vi "Main.vi"(8 "error in (no error)":errorcluster, 11 "ModuleAdmin":refnum<class "ModuleAdmin.lvclass">) -> ()   [LabVIEW 2014, in "SamplerModule.lvlib"]
uses:
  SamplerModule.lvlib
  <userlib>/NIST/ModuleAdminLib/ModuleAdmin/ModuleAdmin.lvclass
  PublicAPI/Arguments/Requests/clStopArgument.ctl
  SamplerPlugins/NISTSamplerPluginsBaseClass/SamplerPluginsBase.lvclass
  <userlib>/NIST/ModuleAdminLib/ModuleAdmin/ModuleAdmin.lvclass/ModuleAdmin.ctl
  <userlib>/NIST/BaseClasses/BasePlugin_class/BasePlugin.lvclass/BasePlugin.ctl
  SamplerPlugins/NISTSamplerPluginsBaseClass/TypeDefs/ConfigMeasurementParams.ctl
  SamplerPlugins/NISTSamplerPluginsBaseClass/TypeDefs/ConfigTriggerParams.ctl
  SamplerPlugins/NISTSamplerPluginsBaseClass/TypeDefs/ConfigACBandwidthParams.ctl
  SamplerPlugins/NISTSamplerPluginsBaseClass/TypeDefs/ConfigMultiPointParams.ctl
  SamplerPlugins/NISTSamplerPluginsBaseClass/TypeDefs/MultiPointParams.ctl
  SamplerPlugins/NISTSamplerPluginsBaseClass/TypeDefs/CorrectionFactors.ctl
  SamplerPlugins/NISTSamplerPluginsBaseClass/SamplerPluginsBase.lvclass/SamplerPluginsBase.ctl
  <vilib>/Utility/error.llb/DialogType.ctl
  <userlib>/NIST/ModuleAdminLib/ModuleAdmin/Accessors/Read ShowPanel_.vi
  <userlib>/NIST/BaseClasses/BasePlugin_class/Accessors/Write PluginIniFilePath.vi
  <userlib>/NIST/BaseClasses/BasePlugin_class/Accessors/Read PluginIniFilePath.vi
  SamplerPlugins/NISTSamplerPluginsBaseClass/Accessors/Write CorrectionFactors.vi
  SamplerPlugins/NISTSamplerPluginsBaseClass/Accessors/Read CorrectionFactors.vi
  <userlib>/NIST/ModuleAdminLib/ModuleAdmin/Accessors/Write ShowPanel_.vi
  <userlib>/NIST/ModuleAdminLib/ModuleAdmin/Accessors/Read CloneRegRef.vi
  <vilib>/Utility/error.llb/Error Cluster From Error Code.vi
  <vilib>/ErrorRing/Error Ring.xnode
  <userlib>/NIST/ModuleAdminLib/CloneRegistration/CloneRegistration.lvclass
  <userlib>/NIST/ModuleAdminLib/ModuleAdmin.lvlib
  <userlib>/NIST/BaseClasses/Object_class/BaseObject.lvclass
panel:
  out "error out":errorcluster
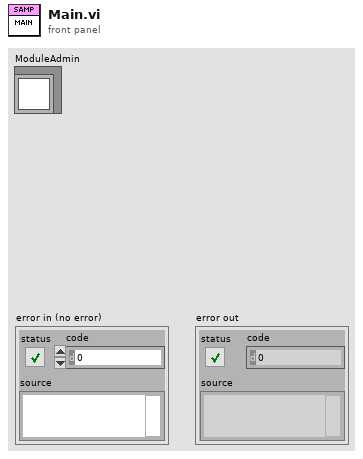
[diagram p1: front panel]
types:
  T1 = typedef "SamplerModule.lvlib/clRequestEvents.ctl" = cluster{"StopRequest":refnum<user-event>, "PathToINI":refnum<user-event>, " LoadPlugin":refnum<user-event>, "ConfigMeasurement":refnum<user-event>, "Read":refnum<user-event>, "GetReading":refnum<user-event>, "InitializeDevice":refnum<user-event>, "ResetRequest":refnum<user-event>, "AbortRequest":refnum<user-event>, "FetchRequest":refnum<user-event>, "InitiateRequest":refnum<user-event>, "ConfigTrigger":refnum<user-event>, "IsOverRange":refnum<user-event>, "ConfigACBandwidth":refnum<user-event>, "ConfigFreqVoltRange":refnum<user-event>, "ConfigMeasCompDest":refnum<user-event>, "FetchMultiPoint":refnum<user-event>, "ReadMultiPoint":refnum<user-event>, "ConfigMultiPoint":refnum<user-event>, "GetMultiPointReading":refnum<user-event>, "InitiateMultiPoint":refnum<user-event>, "ShowPanel":refnum<user-event>, "WriteMultiPointParams":refnum<user-event>, "EvtSignal":refnum<user-event>, "ReadMultiPointParams":refnum<user-event>, "ReadMultiPointConfig":refnum<user-event>, "WriteMultiPointConfig":refnum<user-event>, "ReadCorrFactors":refnum<user-event>, "Write CorrFactors":refnum<user-event>, "ConfigDialog":refnum<user-event>}
  T2 = typedef "SamplerModule.lvlib/clBroadcastEvents.ctl" = cluster{"DidInit":refnum<user-event>, "StatusUpdate":refnum<user-event>, "ErrorReport":refnum<user-event>, "DidStop":refnum<user-event>, "PathToINI":refnum<user-event>, "GetReading":refnum<user-event>, "IsOverRange":refnum<user-event>, "GetMultiPointReading":refnum<user-event>, "MultiPointParams":refnum<user-event>, "MultiPointConfig":refnum<user-event>, "CorrFactors":refnum<user-event>}
  T3 = typedef "SamplerModule.lvlib/clStopArgument.ctl" = cluster{"Exit via Stop Module Req?":bool, "Wait for Module to stop?":bool, "ModuleAdmin":refnum<class "ModuleAdmin.lvclass">}
  T4 = enum32{"Invalid", "Standard", "Closed", "Hidden", "Minimized", "Maximized"}
  T5 = typedef "SamplerPlugins.lvlib/SamplerPluginsBase.lvclass/ConfigMeasurementParams.ctl" = cluster{"eFunction":u16, "dRange":dbl, "dResolution":dbl}
  T6 = typedef "SamplerPlugins.lvlib/SamplerPluginsBase.lvclass/ConfigTriggerParams.ctl" = cluster{"eTriggerSource":u16, "dTriggerDelay":dbl}
  T7 = typedef "SamplerPlugins.lvlib/SamplerPluginsBase.lvclass/ConfigACBandwidthParams.ctl" = cluster{"dMinFreq":dbl, "dMaxFreq":dbl}
  T8 = typedef "SamplerPlugins.lvlib/SamplerPluginsBase.lvclass/ConfigMultiPointParams.ctl" = cluster{"iTriggerCount":i32, "iSampleCount":i32, "eSampleClock":u16, "dSampleInterval":dbl}
  T9 = typedef "SamplerPlugins.lvlib/SamplerPluginsBase.lvclass/MultiPointParams.ctl" = cluster{"iMaxTimeMilliseconds":i32, "iArraySize":i32}
  T10 = typedef "SamplerPlugins.lvlib/SamplerPluginsBase.lvclass/CorrectionFactors.ctl" = cluster{"MagCorr":dbl[], "DlyCorr":dbl[]}
  T11 = typedef "SamplerPlugins.lvlib/SamplerPluginsBase.lvclass/MultiPointReadingArrayParams.ctl" = T12[]
  T12 = typedef "SamplerPlugins.lvlib/SamplerPluginsBase.lvclass/MultiPointReadingParams.ctl" = cluster{"dReadingArray":dbl[], "iActualPts":i32, "Timestamp":dbl}
  T13 = typedef "DialogType.ctl" = u16
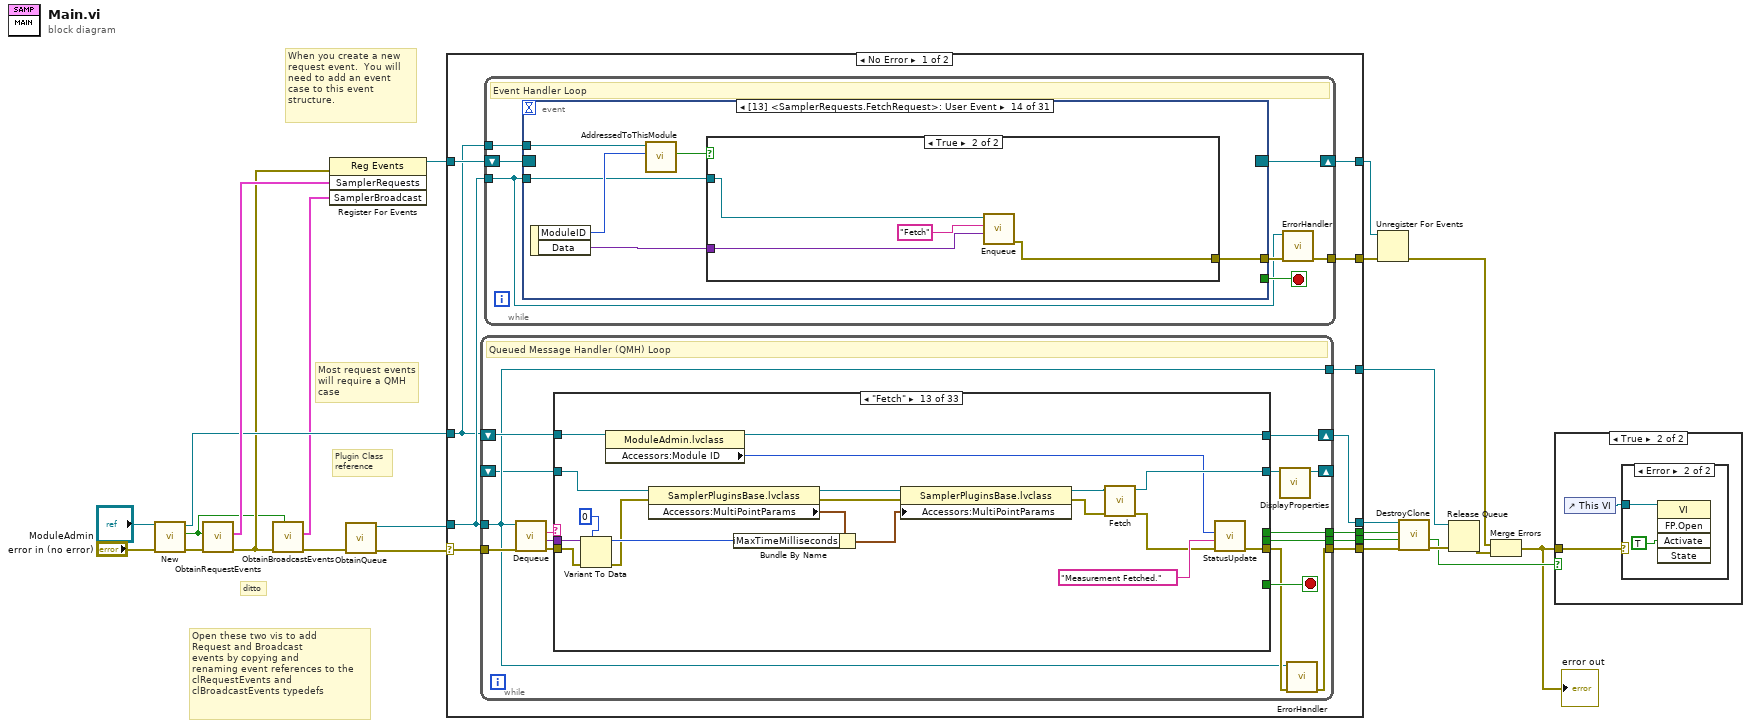
[diagram p0: block diagram]
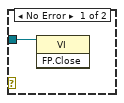
[diagram p3: hidden frame]
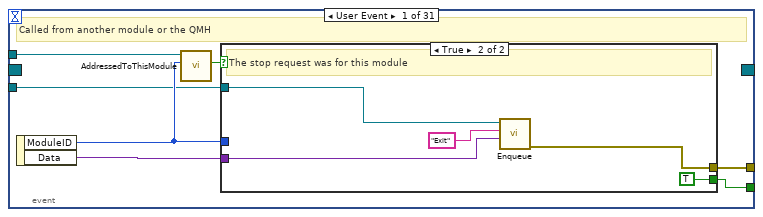
[diagram p4: hidden frame]
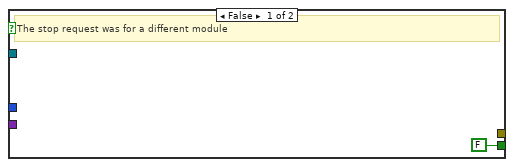
[diagram p5: hidden frame]
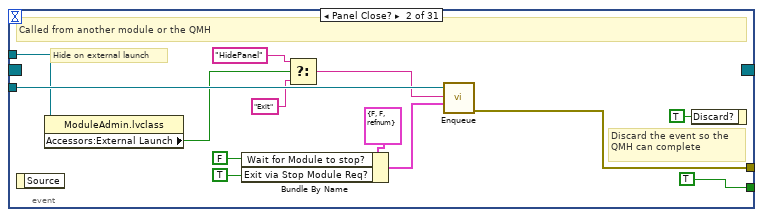
[diagram p6: hidden frame]
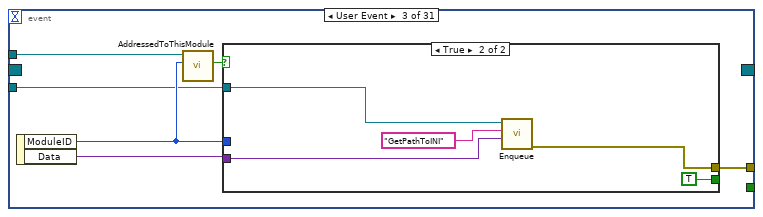
[diagram p7: hidden frame]
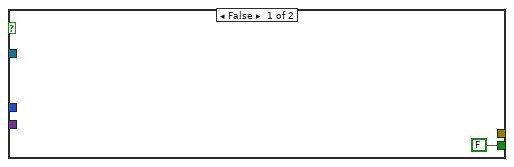
[diagram p8: hidden frame]
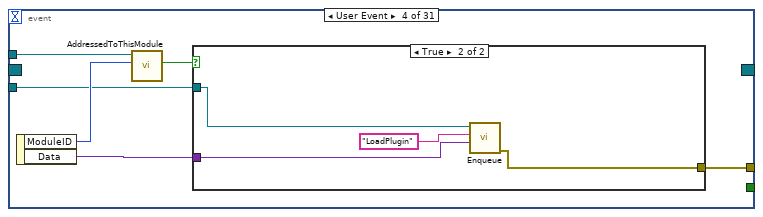
[diagram p9: hidden frame]
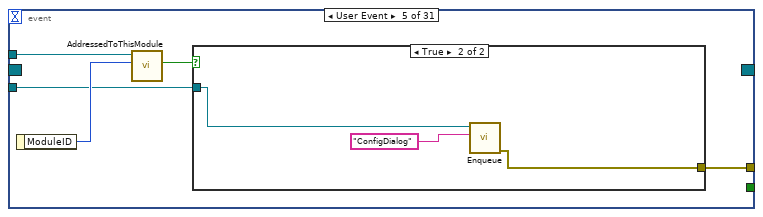
[diagram p11: hidden frame]
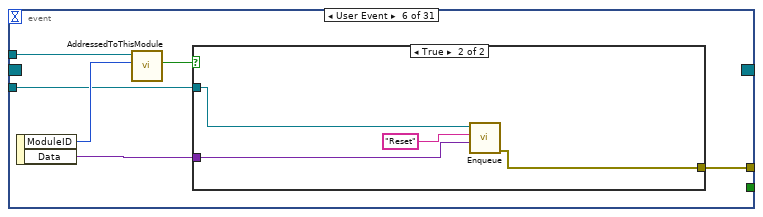
[diagram p13: hidden frame]
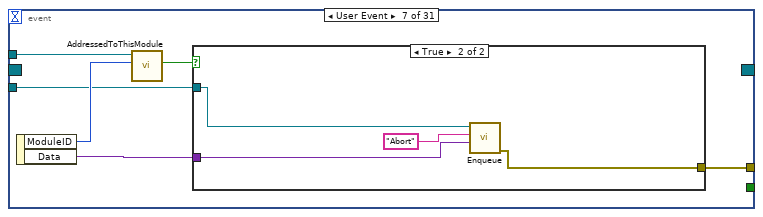
[diagram p15: hidden frame]
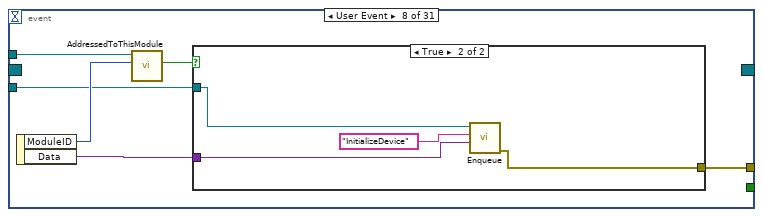
[diagram p17: hidden frame]
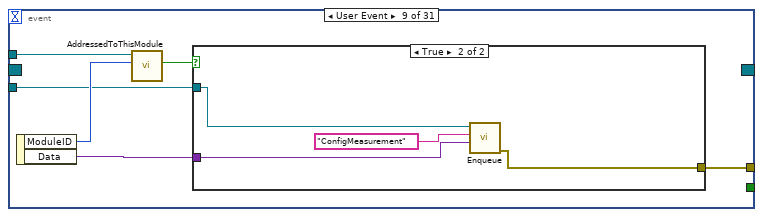
[diagram p19: hidden frame]
diagram:
  # "Plugin Class\nreference"
  # "Open these two vis to add\nRequest and Broadcast \nevents by copying and \nrenaming event references to the \nclRequestEvents and \nclBroadcastEvents typedefs"
  # "ditto"
  # "Most request events\nwill require a QMH\ncase"
  # "When you create a new request event.  You will need to add an event case to this event structure."
  n1 = call <userlib>:"New.vi"("error in (no error)"="error in (no error)", "ModuleAdmin"="ModuleAdmin") -> ("error out"=w22:errorcluster, "First?"=w1:bool, "ModuleAdmin"=w18:refnum<class "ModuleAdmin.lvclass">)  [unwired: 7 in]
  n2 = call "ObtainRequestEvents.vi"("error in (no error)"=w22, "CreateNew (f)"=w1) -> ("error out"=w15:errorcluster, "SamplerRequests"=w21:T1)  [unwired: 8 in]
  n3 = call "ObtainBroadcastEvents.vi"("Init? (f)"=w1, "error in (no error)"=w15) -> ("error out"=w16:errorcluster, "SamplerBroadcast"=w14:T2)  [unwired: 8 in]
  n4 = register-events(error in=w15, w21, w14) -> (reference out=w13:refnum<event-registration>)  [unwired: 1 in, 1 out]
  n5 = call "ObtainQueue.vi"("error in (no error)"=w16) -> ("error out"=w20:errorcluster, "MessageQueue"=w19:refnum<queue>)  [unwired: 9 in]
  n6 = case shown="No Error" w20 {
    selector: w20 -> [w35 w866]
    tunnel: w19 -> [w33 w862]
    tunnel: w18 -> [w30 w863]
    tunnel: [w34 w864] -> w12
    tunnel: [w32 w862] -> w17
    tunnel: w13 -> [w31 w858]
    tunnel: [w29 w861] -> w10
    tunnel: [w28 _] -> w9
    tunnel: [w27 _] -> w8
    tunnel: [w26 _] -> w5
    tunnel: [w25 w858] -> w4
    frame No Error {
      n7 = while {
        tunnel: w33 -> [w361]
        tunnel: w35 -> [w370]
        tunnel: [w363] -> w34
        tunnel: [w361] -> w32
        tunnel: [w365] -> w28
        tunnel: [w364] -> w27
        shift-right: [w358] -> _
        shift-left: _ -> [w360]
        shift-right: [w357] -> w29
        shift-left: w30 -> [w366]
        stop <- w371 stop-if-true
        # "Queued Message Handler (QMH) Loop"
        n8 = call "Dequeue.vi"("error in (no error)"=w370, "MessageQueue"=w361) -> ("error out"=w369:errorcluster, "Message Data"=w367:variant, "Message"=w368:string)  [unwired: 6 in, 1 out]
        n9 = case shown="\"Fetch\"" w368 {
          selector: w368 -> [w376 _ _ _ _ _ _ _ _ _ _ _ _ _ _ _ _ _ _ _ _ _ _ _ _ _ _ _ _ _ _ _ _]
          tunnel: [_ _ _ _ _ _ _ _ _ _ _ _ _ _ TRUE _ _ _ _ _ _ _ _ _ _ _ _ _ _ _ _ _ _] -> w371
          tunnel: w366 -> [w379 w408 w425 w434 w443 w453 w493 w503 w524 w542 w557 w572 w592 w604 w605 w625 w648 w659 w675 w686 w702 w717 w730 w747 w756 w765 w785 w798 w810 w820 w830 w839 w848]
          tunnel: [w375 w397 w424 w433 w442 w454 w492 w501 w523 w541 w556 w571 w591 w603 w614 w626 w649 w655 w668 w684 w701 w716 w729 w746 w755 w764 w784 w797 w803 w814 w824 w836 w851] -> w362
          tunnel: w369 -> [_ _ w421 w431 w440 w458 w496 w512 w530 w545 w560 w575 w594 w600 w607 w634 w644 w656 w672 w678 w705 w720 w726 w742 w751 w768 w788 w801 w811 w821 w831 w843 w849]
          tunnel: w367 -> [_ _ _ _ _ w460 _ w513 w531 w546 w561 w576 w595 _ w613 w633 _ _ _ _ w706 w721 _ _ _ w769 w789 w802 _ _ _ w845 w850]
          tunnel: [_ _ _ _ _ _ _ _ _ _ _ _ _ _ w611 _ _ _ _ _ _ _ _ _ _ _ _ _ _ _ _ _ _] -> w365
          tunnel: [_ _ _ _ _ _ _ _ _ _ _ _ _ _ w610 _ _ _ _ _ _ _ _ _ _ _ _ _ _ _ _ _ _] -> w364
          tunnel: [w373 refnum<class "SamplerPluginsBase.lvclass"> refnum ("MyPlugins.lvlib:MyPluginsBase.lvclass") w423 w430 w441 w451 w494 w502 w521 w540 w555 w568 w587 w601 w608 w624 w645 w657 w673 w685 w688 w711 w727 w740 w754 w761 w781 w794 w805 w816 w826 w840 w846] -> w359
          tunnel: w360 -> [w373 _ w422 w432 w439 w452 w495 w511 w529 w544 w559 w574 w593 w602 w609 w624 w647 w658 w674 w680 w704 w719 w728 w743 w753 w767 w787 w800 w812 w822 w832 w842 w846]
          tunnel: [w372 w392 w420 w429 w438 w450 w493 w500 w518 w535 w550 w565 w586 w599 w605 w622 w642 w651 w670 w676 w687 w710 w725 w744 w752 w760 w780 w793 w806 w817 w827 w838 w847] -> w357
          frame Default {
            # "Called only if a message was queued and no QMH case was created"
            n10 = property class="ModuleAdmin.lvclass"(reference=w379) -> (reference out=w372:refnum<class "ModuleAdmin.lvclass">, "Accessors:Module ID"=w378:i32, "Accessors:ModuleName"=w374:string)  [unwired: 1 in, 1 out]
            n11 = call <userlib>:"ModuleName.vi"("Name"=w374, "ModuleID"=w378) -> ("ModuleName"=w377:string)  [unwired: 9 in]
            n12 = xnode "Error Ring"("parameter 0"=w376, "parameter 1"=w377) -> ("error out"=w375:errorcluster)
          }
          frame "Initialize" {
            # "Initialize is always called after ObtainQueue.vi is run"
            n13 = property class="ModuleAdmin.lvclass"(reference=w408) -> (reference out=w394:refnum<class "ModuleAdmin.lvclass">, error out=w405:errorcluster, "Accessors:Module ID"=w396:i32, "Accessors:ShowPanel_"=w391:bool, "Accessors:External Launch"=w389:bool, "Accessors:ModuleName"=w388:string)  [unwired: 1 in]
            n14 = Compound Arithmetic op=OR(w391, invert w389) -> (w390:bool)
            n15 = Select(t=T4."Standard" ("Front Panel Window:State"), s=w390, f=T4."Hidden" ("Front Panel Window:State")) -> (s? t:f=w401:T4)
            n16 = invoke class="VI" method="FP.Open"(error in=w405, "State"=w401) -> (error out=w404:errorcluster)  [unwired: 3 in, 4 out]
            n17 = call <userlib>:"ModuleName.vi"("Name"=w388, "ModuleID"=w396) -> ("ModuleName"=w400:string)  [unwired: 9 in]
            n18 = property class="VI"(error in=w404, "Front Panel.Title"=w400) -> (reference out=w407:refnum<vi>, error out=w406:errorcluster)  [unwired: 1 in]
            n19 = invoke class="VI" method="FP.Center"(reference=w407, error in=w406) -> (error out=w395:errorcluster)  [unwired: 1 in, 2 out]
            n20 = case shown="True" w389 {
              tunnel: [w409 w415] -> w398
              tunnel: [w410 w412] -> w392
              tunnel: w395 -> [w409 w414]
              tunnel: w394 -> [w410 w411]
              frame False {
              }
              frame True {
                n21 = call <userlib>:"WaitOnModuleSync.vi"("error in (no error)"=w414, "ModuleAdmin"=w411) -> ("error out"=w416:errorcluster, "ModuleAdmin"=w413:refnum<class "ModuleAdmin.lvclass">)  [unwired: 8 in]
                n22 = call <userlib>:"WaitOnEventSync.vi"("error in (no error)"=w416, "ModuleAdmin"=w413) -> ("error out"=w415:errorcluster, "ModuleAdmin"=w412:refnum<class "ModuleAdmin.lvclass">)  [unwired: 8 in]
              }
            }
            n23 = call "DidInit.vi"("Init?"=TRUE, "error in (no error)"=w398, "ModuleAdmin"=w392) -> ("error out"=w397:errorcluster)  [unwired: 8 in]
          }
          frame "Reset" {
            n24 = property class="ModuleAdmin.lvclass"(reference=w425) -> (reference out=w420:refnum<class "ModuleAdmin.lvclass">, "Accessors:Module ID"=w417:i32)  [unwired: 1 in, 1 out]
            n25 = call-dynamic "Reset.vi"("error in (no error)"=w421, "NISTSamplerPluginsBase in"=w422) -> ("error out"=w418:errorcluster, "NISTSamplerPluginsBase out"=w423:refnum<class "SamplerPluginsBase.lvclass">)  [unwired: 8 in]
            n26 = call "StatusUpdate.vi"("error in (no error)"=w418, "Status"="Device is reset.", "ModuleID"=w417) -> ("error out"=w424:errorcluster)  [unwired: 8 in]
          }
          frame "Abort" {
            n27 = property class="ModuleAdmin.lvclass"(reference=w434) -> (reference out=w429:refnum<class "ModuleAdmin.lvclass">, "Accessors:Module ID"=w427:i32)  [unwired: 1 in, 1 out]
            n28 = call-dynamic "Abort.vi"("error in (no error)"=w431, "NISTSamplerPluginsBase in"=w432) -> ("error out"=w428:errorcluster, "NISTSamplerPluginsBase out"=w430:refnum<class "SamplerPluginsBase.lvclass">)  [unwired: 8 in]
            n29 = call "StatusUpdate.vi"("error in (no error)"=w428, "Status"="Operation Aborted.", "ModuleID"=w427) -> ("error out"=w433:errorcluster)  [unwired: 8 in]
          }
          frame "InitializeDevice" {
            # "Resets the device, clear tasks, creates new task, sets trigger and clock"
            n30 = property class="ModuleAdmin.lvclass"(reference=w443) -> (reference out=w438:refnum<class "ModuleAdmin.lvclass">, "Accessors:Module ID"=w437:i32)  [unwired: 1 in, 1 out]
            n31 = call-dynamic "InitializeDevice.vi"("error in (no error)"=w440, "NISTSamplerPluginsBase in"=w439) -> ("error out"=w435:errorcluster, "NISTSamplerPluginsBase out"=w441:refnum<class "SamplerPluginsBase.lvclass">)  [unwired: 8 in]
            n32 = call "StatusUpdate.vi"("error in (no error)"=w435, "Status"="Device is initialized.", "ModuleID"=w437) -> ("error out"=w442:errorcluster)  [unwired: 8 in]
          }
          frame "LoadPlugin" {
            n33 = Variant To Data(error in=w458, type=path "", Variant=w460) -> (data=w448:path, error out=w449:errorcluster)
            n34 = call <userlib>:"GetPathToClass.vi"("error in (no error)"=w449, "configuration file path"=w448) -> ("error IO"=w445:errorcluster, "PathToClass"=w447:path)  [unwired: 8 in]
            n35 = Current VI's Path() -> (path=w446:path)
            n36 = Build Path(base path=w446, name or relative path=w447) -> (appended path=w444:path)
            n37 = call <vilib>:"Check if File or Folder Exists.vi"("error in (no error)"=w445, "path"=w444) -> ("error out"=w455:errorcluster, "file or folder exists?"=w457:bool, "dup path"=w456:path)  [unwired: 7 in]
            n38 = case shown="True" w457 {
              tunnel: w456 -> [w466 w483]
              tunnel: w455 -> [w464 w491]
              tunnel: [w462 w486] -> w454
              tunnel: w453 -> [w461 w485]
              tunnel: w452 -> [w465 _]
              tunnel: [w465 w476] -> w451
              tunnel: w448 -> [_ w482]
              tunnel: [w461 w481] -> w450
              frame False {
                n39 = Path To String(path=w466) -> (string=w467:string)
                n40 = xnode "Error Ring"("parameter 0"=w467) -> ("error out"=w463:errorcluster)
                n41 = Merge Errors(w464, w463) -> (w462:errorcluster)
              }
              frame True {
                n42 = call-dynamic "LoadClassFromFile.vi"("error in (no error)"=w491, "class path"=w483, "reference in"=refnum<class "SamplerPluginsBase.lvclass"> refnum ("MyPlugins.lvlib:MyPluginsBase.lvclass")) -> ("error out"=w480:errorcluster, "reference out"=w479:refnum<class "SamplerPluginsBase.lvclass">)  [unwired: 7 in]
                n43 = property class="SamplerPluginsBase.lvclass"(reference=w479, error in=w480, "Accessors:PluginIniFilePath"=w482) -> (reference out=w478:refnum<class "SamplerPluginsBase.lvclass">, error out=w477:errorcluster)
                n44 = property class="ModuleAdmin.lvclass"(reference=w485) -> (reference out=w481:refnum<class "ModuleAdmin.lvclass">, "Accessors:Module ID"=w484:i32)  [unwired: 1 in, 1 out]
                n45 = Path To String(path=w483) -> (string=w488:string)
                n46 = Format Into String(format string="Plugin %s loaded ", w488) -> (resulting string=w487:string)  [unwired: 2 in, 1 out]
                n47 = call-dynamic "DefaultFromIni.vi"("error in (no error)"=w477, "SamplerPluginsBase in"=w478) -> ("error out"=w475:errorcluster, "SamplerPluginsBase out"=w476:refnum<class "SamplerPluginsBase.lvclass">)  [unwired: 8 in]
                n48 = call "StatusUpdate.vi"("error in (no error)"=w475, "Status"=w487, "ModuleID"=w484) -> ("error out"=w486:errorcluster)  [unwired: 8 in]
              }
            }
          }
          frame "ConfigDialog" {
            n49 = call-dynamic "ConfigDialog.vi"("error in (no error)"=w496, "SamplerPluginsBase in"=w495) -> ("error out"=w492:errorcluster, "SamplerPluginsBase out"=w494:refnum<class "SamplerPluginsBase.lvclass">)  [unwired: 8 in]
          }
          frame "ConfigMeasurement" {
            n50 = Variant To Data(error in=w512, type=T5 {"eFunction"=0, "dRange"=0.0, "dResolution"=0.0} ("ConfigMeasurement"), Variant=w513) -> (data=w510:T5, error out=w505:errorcluster)
            n51 = property class="ModuleAdmin.lvclass"(reference=w503) -> (reference out=w500:refnum<class "ModuleAdmin.lvclass">, "Accessors:Module ID"=w497:i32)  [unwired: 1 in, 1 out]
            n52 = Unbundle By Name(w510) -> ("eFunction"=w509:u16, "dRange"=w508:dbl, "dResolution"=w507:dbl)
            n53 = property class="SamplerPluginsBase.lvclass"(reference=w511, error in=w505, "Accessors:eFunction"=w509, "Accessors:dRange"=w508, "Accessors:dResolution"=w507) -> (reference out=w506:refnum<class "SamplerPluginsBase.lvclass">, error out=w504:errorcluster)
            n54 = call-dynamic "ConfigMeasurement.vi"("error in (no error)"=w504, "NISTSamplerPluginsBase in"=w506) -> ("error out"=w499:errorcluster, "NISTSamplerPluginsBase out"=w502:refnum<class "SamplerPluginsBase.lvclass">)  [unwired: 8 in]
            n55 = call "StatusUpdate.vi"("error in (no error)"=w499, "Status"="Measurement Configured." ("input 3"), "ModuleID"=w497) -> ("error out"=w501:errorcluster)  [unwired: 8 in]
          }
          frame "ConfigTrigger" {
            n56 = Variant To Data(error in=w530, type=T6 {"eTriggerSource"=0, "dTriggerDelay"=0.0} ("ConfigTriggerParams"), Variant=w531) -> (data=w528:T6, error out=w525:errorcluster)
            n57 = property class="ModuleAdmin.lvclass" props=["Accessors:Module ID", "Accessors:Module ID"](reference=w524) -> (reference out=w518:refnum<class "ModuleAdmin.lvclass">, "Accessors:Module ID"=w517:i32)  [unwired: 1 in, 2 out]
            n58 = Unbundle By Name(w528) -> ("eTriggerSource"=w527:u16, "dTriggerDelay"=w526:dbl)
            n59 = property class="SamplerPluginsBase.lvclass"(reference=w529, error in=w525, "Accessors:eTriggerSource"=w527, "Accessors:dTriggerDelay"=w526) -> (reference out=w520:refnum<class "SamplerPluginsBase.lvclass">, error out=w519:errorcluster)
            n60 = call-dynamic "ConfigTrigger.vi"("error in (no error)"=w519, "NISTSamplerPluginsBase in"=w520) -> ("error out"=w516:errorcluster, "NISTSamplerPluginsBase out"=w521:refnum<class "SamplerPluginsBase.lvclass">)  [unwired: 8 in]
            n61 = call "StatusUpdate.vi"("error in (no error)"=w516, "Status"="Trigger Configured." ("input 3"), "ModuleID"=w517) -> ("error out"=w523:errorcluster)  [unwired: 8 in]
          }
          frame "ConfigACBandwidth" {
            n62 = Variant To Data(error in=w545, type=T7 {"dMinFreq"=0.0, "dMaxFreq"=0.0} ("ConfigACBandwidthParams"), Variant=w546) -> (data=w537:T7, error out=w543:errorcluster)
            n63 = property class="ModuleAdmin.lvclass"(reference=w542) -> (reference out=w535:refnum<class "ModuleAdmin.lvclass">, "Accessors:Module ID"=w534:i32)  [unwired: 1 in, 1 out]
            n64 = property class="SamplerPluginsBase.lvclass"(reference=w544, error in=w543, "Accessors:ConfigACBandwidthParams"=w537) -> (reference out=w539:refnum<class "SamplerPluginsBase.lvclass">, error out=w536:errorcluster)
            n65 = call-dynamic "ConfigACBandwidth.vi"("error in (no error)"=w536, "NISTSamplerPluginsBase in"=w539) -> ("error out"=w533:errorcluster, "NISTSamplerPluginsBase out"=w540:refnum<class "SamplerPluginsBase.lvclass">)  [unwired: 8 in]
            n66 = call "StatusUpdate.vi"("error in (no error)"=w533, "Status"="AC Bandwidth Configured." ("input 3"), "ModuleID"=w534) -> ("error out"=w541:errorcluster)  [unwired: 8 in]
          }
          frame "ConfigFreqVoltRange" {
            n67 = Variant To Data(error in=w560, type=0.0 ("dFrequencyVoltageRange"), Variant=w561) -> (data=w551:dbl, error out=w558:errorcluster)
            n68 = property class="ModuleAdmin.lvclass" props=["Accessors:Module ID", "Accessors:Module ID"](reference=w557) -> (reference out=w550:refnum<class "ModuleAdmin.lvclass">, "Accessors:Module ID"=w549:i32)  [unwired: 1 in, 2 out]
            n69 = property class="SamplerPluginsBase.lvclass"(reference=w559, error in=w558, "Accessors:dFrequencyVoltageRange"=w551) -> (reference out=w553:refnum<class "SamplerPluginsBase.lvclass">, error out=w554:errorcluster)
            n70 = call-dynamic "ConfigFreqVoltRange.vi"("error in (no error)"=w554, "NISTSamplerPluginsBase in"=w553) -> ("error out"=w548:errorcluster, "NISTSamplerPluginsBase out"=w555:refnum<class "SamplerPluginsBase.lvclass">)  [unwired: 8 in]
            n71 = call "StatusUpdate.vi"("error in (no error)"=w548, "Status"="Frequency Voltage Range Configured." ("input 3"), "ModuleID"=w549) -> ("error out"=w556:errorcluster)  [unwired: 8 in]
          }
          frame "Read" {
            n72 = Variant To Data(error in=w575, type=0 ("iMaxTimeMilliseconds"), Variant=w576) -> (data=w570:i32, error out=w573:errorcluster)
            n73 = property class="ModuleAdmin.lvclass"(reference=w572) -> (reference out=w565:refnum<class "ModuleAdmin.lvclass">, "Accessors:Module ID"=w564:i32)  [unwired: 1 in, 1 out]
            n74 = property class="SamplerPluginsBase.lvclass"(reference=w574, error in=w573, "Accessors:iMaxTimeMilliseconds"=w570) -> (reference out=w566:refnum<class "SamplerPluginsBase.lvclass">, error out=w567:errorcluster)
            n75 = call-dynamic "Read.vi"("error in (no error)"=w567, "NISTSamplerPluginsBase in"=w566) -> ("error out"=w562:errorcluster, "NISTSamplerPluginsBase out"=w568:refnum<class "SamplerPluginsBase.lvclass">)  [unwired: 8 in]
            n76 = call "StatusUpdate.vi"("error in (no error)"=w562, "Status"="Measurement Read." ("input 3"), "ModuleID"=w564) -> ("error out"=w571:errorcluster)  [unwired: 8 in]
          }
          frame "Fetch" {
            n77 = Variant To Data(error in=w594, type=0 ("iMaxTimeMilliseconds"), Variant=w595) -> (data=w582:i32, error out=w580:errorcluster)
            n78 = property class="ModuleAdmin.lvclass"(reference=w592) -> (reference out=w586:refnum<class "ModuleAdmin.lvclass">, "Accessors:Module ID"=w585:i32)  [unwired: 1 in, 1 out]
            n79 = property class="SamplerPluginsBase.lvclass"(reference=w593, error in=w580) -> (reference out=w581:refnum<class "SamplerPluginsBase.lvclass">, error out=w579:errorcluster, "Accessors:MultiPointParams"=w578:T9)
            n80 = Bundle By Name(cluster=w578, "iMaxTimeMilliseconds"=w582) -> (w577:T9)
            n81 = property class="SamplerPluginsBase.lvclass"(reference=w581, error in=w579, "Accessors:MultiPointParams"=w577) -> (reference out=w589:refnum<class "SamplerPluginsBase.lvclass">, error out=w588:errorcluster)
            n82 = call-dynamic "Fetch.vi"("error in (no error)"=w588, "NISTSamplerPluginsBase in"=w589) -> ("error out"=w583:errorcluster, "NISTSamplerPluginsBase out"=w587:refnum<class "SamplerPluginsBase.lvclass">)  [unwired: 8 in]
            n83 = call "StatusUpdate.vi"("error in (no error)"=w583, "Status"="Measurement Fetched." ("input 3"), "ModuleID"=w585) -> ("error out"=w591:errorcluster)  [unwired: 8 in]
          }
          frame "Initiate" {
            n84 = property class="ModuleAdmin.lvclass"(reference=w604) -> (reference out=w599:refnum<class "ModuleAdmin.lvclass">, "Accessors:Module ID"=w598:i32)  [unwired: 1 in, 1 out]
            n85 = call-dynamic "Initiate.vi"("error in (no error)"=w600, "NISTSamplerPluginsBase in"=w602) -> ("error out"=w596:errorcluster, "NISTSamplerPluginsBase out"=w601:refnum<class "SamplerPluginsBase.lvclass">)  [unwired: 8 in]
            n86 = call "StatusUpdate.vi"("error in (no error)"=w596, "Status"="Measurement Initiated.", "ModuleID"=w598) -> ("error out"=w603:errorcluster)  [unwired: 8 in]
          }
          frame "Exit" {
            # "Called by the StopRequest event handler case"
            n87 = disable-structure shown="Enabled" {
              disable-tunnel: w609 -> [w619 w621]
              disable-tunnel: [w618 w621] -> w608
              disable-tunnel: w607 -> [w617 w620]
              disable-tunnel: [w616 w620] -> w606
              frame Enabled {
                n88 = call-dynamic "CloseInstrumentSession.vi"("error in (no error)"=w617, "NISTSamplerPluginsBase in"=w619) -> ("error out"=w616:errorcluster, "NISTSamplerPluginsBase out"=w618:refnum<class "SamplerPluginsBase.lvclass">)  [unwired: 8 in]
              }
              frame Disabled {
              }
            }
            n89 = control-ref of="This VI"() -> (w612:refnum<vi>)
            n90 = call "HandleExit.vi"("error in (no error)"=w606, "VI Refnum"=w612, "StopArgument"=w613, "ModuleAdmin"=w605) -> ("error out"=w614:errorcluster, "Exit via Stop Module Req?"=w610:bool, "WaitForStop?"=w611:bool)  [unwired: 5 in]
          }
          frame "Error" {
            n91 = property class="ModuleAdmin.lvclass"(reference=w625) -> (reference out=w623:refnum<class "ModuleAdmin.lvclass">, "Accessors:External Launch"=w629:bool, "Accessors:Module ID"=w627:i32)  [unwired: 1 in, 1 out]
            n92 = Variant To Data(error in=w634, type=errorcluster {"status"=FALSE, "code"=0, "source"=""} ("error constant"), Variant=w633) -> (data=w628:errorcluster, error out=w631:errorcluster)
            n93 = call "ReportError.vi"("error in (no error)"=w631, "ErrorReported"=w628, "ModuleID"=w627) -> ("error out"=w630:errorcluster)  [unwired: 8 in]
            n94 = case shown="True" w629 {
              tunnel: w630 -> [w639 w641]
              tunnel: w628 -> [w638 _]
              tunnel: [w637 w641] -> w626
              tunnel: w625 -> [w636 _]
              tunnel: w623 -> [w635 w640]
              tunnel: [w635 w640] -> w622
              frame False {
                # "Todo:  Add an event to ask the user\nIf the module should stop or continue"
                # "Stand alone: now, force an exit"
                n95 = call <vilib>:"Simple Error Handler.vi"("error in (no error)"=w638) -> ()  [unwired: 4 in, 5 out]
                n96 = call "StopRequest.vi"("error in (no error)"=w639, "ModuleAdmin"=w636) -> ("error out"=w637:errorcluster)  [unwired: 8 in, 1 out]
              }
              frame True {
                # "Externally launched modules only broadcast the error msg"
              }
            }
          }
          frame "GetPathToINI" {
            n97 = property class="SamplerPluginsBase.lvclass"(reference=w647, error in=w644) -> (reference out=w645:refnum<class "SamplerPluginsBase.lvclass">, error out=w643:errorcluster, "Accessors:PluginIniFilePath"=w646:path)
            n98 = property class="ModuleAdmin.lvclass"(reference=w648) -> (reference out=w642:refnum<class "ModuleAdmin.lvclass">, "Accessors:Module ID"=w650:i32)  [unwired: 1 in, 1 out]
            n99 = call "PathToINIBroadcast.vi"("error in (no error)"=w643, "PathToINI"=w646, "ModuleID"=w650) -> ("error out"=w649:errorcluster)  [unwired: 8 in]
          }
          frame "GetReading" {
            n100 = property class="SamplerPluginsBase.lvclass"(reference=w658, error in=w656) -> (reference out=w657:refnum<class "SamplerPluginsBase.lvclass">, error out=w654:errorcluster, "Accessors:dReading"=w652:dbl[])
            n101 = property class="ModuleAdmin.lvclass"(reference=w659) -> (reference out=w651:refnum<class "ModuleAdmin.lvclass">, "Accessors:Module ID"=w653:i32)  [unwired: 1 in, 1 out]
            n102 = call "GetReadingBroadcast.vi"("error in (no error)"=w654, "dReadingArray"=w652, "ModuleID"=w653) -> ("error out"=w655:errorcluster)  [unwired: 8 in]
          }
          frame "GetMultiPointReading" {
            n103 = property class="SamplerPluginsBase.lvclass"(reference=w674, error in=w672) -> (reference out=w673:refnum<class "SamplerPluginsBase.lvclass">, error out=w671:errorcluster, "Accessors:MultiPointReadingArray"=w667:T11)
            n104 = property class="ModuleAdmin.lvclass"(reference=w675) -> (reference out=w670:refnum<class "ModuleAdmin.lvclass">, "Accessors:Module ID"=w661:i32)  [unwired: 1 in, 1 out]
            n105 = Index Array(array=w667, index=0) -> (element=w666:T12)
            n106 = call "GetMultiPointReadingBroadcast.vi"("error in (no error)"=w671, "MultiPointReadingArray"=w667, "ModuleID"=w661) -> ("error out"=w669:errorcluster)  [unwired: 8 in]
            n107 = Unbundle By Name(w666) -> ("iActualPts"=w664:i32)
            n108 = Format Into String(format string="%d samples", initial string="Transmitted ", w664) -> (resulting string=w662:string)  [unwired: 1 in, 1 out]
            n109 = call "StatusUpdate.vi"("error in (no error)"=w669, "Status"=w662, "ModuleID"=w661) -> ("error out"=w668:errorcluster)  [unwired: 8 in]
          }
          frame "IsOverRange" {
            n110 = call-dynamic "IsOverRange.vi"("error in (no error)"=w678, "NISTSamplerPluginsBase in"=w680) -> ("error out"=w677:errorcluster, "NISTSamplerPluginsBase out"=w679:refnum<class "SamplerPluginsBase.lvclass">)  [unwired: 8 in]
            n111 = property class="ModuleAdmin.lvclass"(reference=w686) -> (reference out=w676:refnum<class "ModuleAdmin.lvclass">, "Accessors:Module ID"=w681:i32)  [unwired: 1 in, 1 out]
            n112 = property class="SamplerPluginsBase.lvclass"(reference=w679, error in=w677) -> (reference out=w685:refnum<class "SamplerPluginsBase.lvclass">, error out=w683:errorcluster, "Accessors:bIsOverRange"=w682:bool)
            n113 = call "IsOverRangeBroadcast.vi"("error in (no error)"=w683, "bIsOverRange"=w682, "ModuleID"=w681) -> ("error out"=w684:errorcluster)  [unwired: 8 in]
          }
          frame "ConfigMeasCompDest" {
            n114 = Variant To Data(error in=w705, type=u16 0 ("eMeasCompleteDest"), Variant=w706) -> (data=w692:u16, error out=w703:errorcluster)
            n115 = property class="ModuleAdmin.lvclass"(reference=w702) -> (reference out=w687:refnum<class "ModuleAdmin.lvclass">, "Accessors:ModuleName"=w696:string, "Accessors:Module ID"=w695:i32)  [unwired: 1 in, 1 out]
            n116 = property class="SamplerPluginsBase.lvclass"(reference=w704, error in=w703, "Accessors:eMeasCompleteDest"=w692) -> (reference out=w689:refnum<class "SamplerPluginsBase.lvclass">, error out=w690:errorcluster)
            n117 = call-dynamic "ConfigMeasCompDest.vi"("error in (no error)"=w690, "NISTSamplerPluginsBase in"=w689) -> ("error out"=w691:errorcluster, "NISTSamplerPluginsBase out"=w688:refnum<class "SamplerPluginsBase.lvclass">)  [unwired: 8 in]
            n118 = Format Into String(format string="%s:%d: %s", initial string="", error in=w691, w696, w695, "Measurement Complete Destination Configured." ("input 3")) -> (resulting string=w699:string, error out=w698:errorcluster)
            n119 = call "StatusUpdate.vi"("error in (no error)"=w698, "Status"=w699, "ModuleID"=w695) -> ("error out"=w701:errorcluster)  [unwired: 8 in]
          }
          frame "ConfigMultiPoint" {
            n120 = Variant To Data(error in=w720, type=T8 {"iTriggerCount"=0, "iSampleCount"=0, "eSampleClock"=0, "dSampleInterval"=0.0} ("ConfigMultiPointParams"), Variant=w721) -> (data=w714:T8, error out=w718:errorcluster)
            n121 = property class="ModuleAdmin.lvclass"(reference=w717) -> (reference out=w710:refnum<class "ModuleAdmin.lvclass">, "Accessors:Module ID"=w709:i32)  [unwired: 1 in, 1 out]
            n122 = property class="SamplerPluginsBase.lvclass"(reference=w719, error in=w718, "Accessors:ConfigMultiPointParams"=w714) -> (reference out=w712:refnum<class "SamplerPluginsBase.lvclass">, error out=w713:errorcluster)
            n123 = call-dynamic "ConfigMultiPoint.vi"("error in (no error)"=w713, "NISTSamplerPluginsBase in"=w712) -> ("error out"=w708:errorcluster, "NISTSamplerPluginsBase out"=w711:refnum<class "SamplerPluginsBase.lvclass">)  [unwired: 8 in]
            n124 = call "StatusUpdate.vi"("error in (no error)"=w708, "Status"="Multi-Point Measurement Configured." ("input 3"), "ModuleID"=w709) -> ("error out"=w716:errorcluster)  [unwired: 8 in]
          }
          frame "InitiateMultiPoint" {
            n125 = property class="ModuleAdmin.lvclass"(reference=w730) -> (reference out=w725:refnum<class "ModuleAdmin.lvclass">, "Accessors:Module ID"=w724:i32)  [unwired: 1 in, 1 out]
            n126 = call-dynamic "InitiateMultiPoint.vi"("error in (no error)"=w726, "NISTSamplerPluginsBase in"=w728) -> ("error out"=w723:errorcluster, "NISTSamplerPluginsBase out"=w727:refnum<class "SamplerPluginsBase.lvclass">)  [unwired: 8 in]
            n127 = call "StatusUpdate.vi"("error in (no error)"=w723, "Status"="Multi-Point Measurement Initiated.", "ModuleID"=w724) -> ("error out"=w729:errorcluster)  [unwired: 8 in]
          }
          frame "FetchMultiPoint" {
            n128 = call-dynamic "FetchMultiPoint.vi"("error in (no error)"=w742, "NISTSamplerPluginsBase in"=w743) -> ("error out"=w739:errorcluster, "NISTSamplerPluginsBase out"=w745:refnum<class "SamplerPluginsBase.lvclass">)  [unwired: 8 in]
            n129 = property class="ModuleAdmin.lvclass"(reference=w747) -> (reference out=w744:refnum<class "ModuleAdmin.lvclass">, "Accessors:Module ID"=w741:i32)  [unwired: 1 in, 1 out]
            n130 = property class="SamplerPluginsBase.lvclass"(reference=w745, error in=w739) -> (reference out=w740:refnum<class "SamplerPluginsBase.lvclass">, error out=w733:errorcluster, "Accessors:MultiPointReadingArray"=w737:T11)
            n131 = Index Array(array=w737) -> (element=w736:T12)  [unwired: 1 in]
            n132 = Unbundle By Name(w736) -> ("iActualPts"=w734:i32)
            n133 = Format Into String(format string="%d samples", initial string="Fetched ", error in=w733, w734) -> (resulting string=w732:string, error out=w731:errorcluster)
            n134 = call "StatusUpdate.vi"("error in (no error)"=w731, "Status"=w732, "ModuleID"=w741) -> ("error out"=w746:errorcluster)  [unwired: 8 in]
          }
          frame "ReadMultiPoint" {
            n135 = property class="ModuleAdmin.lvclass"(reference=w756) -> (reference out=w752:refnum<class "ModuleAdmin.lvclass">, "Accessors:Module ID"=w750:i32)  [unwired: 1 in, 1 out]
            n136 = call-dynamic "ReadMultiPoint.vi"("error in (no error)"=w751, "NISTSamplerPluginsBase in"=w753) -> ("error out"=w748:errorcluster, "NISTSamplerPluginsBase out"=w754:refnum<class "SamplerPluginsBase.lvclass">)  [unwired: 8 in]
            n137 = call "StatusUpdate.vi"("error in (no error)"=w748, "Status"="Multi-Point Measurement Read." ("input 3"), "ModuleID"=w750) -> ("error out"=w755:errorcluster)  [unwired: 8 in]
          }
          frame "WriteMultiPointParams" {
            n138 = Variant To Data(error in=w768, type=T9 {"iMaxTimeMilliseconds"=0, "iArraySize"=0} ("ReadMultiPointParams"), Variant=w769) -> (data=w762:T9, error out=w766:errorcluster)
            n139 = property class="ModuleAdmin.lvclass"(reference=w765) -> (reference out=w760:refnum<class "ModuleAdmin.lvclass">, "Accessors:Module ID"=w759:i32)  [unwired: 1 in, 1 out]
            n140 = disable-structure shown="Enabled" {
              disable-tunnel: w767 -> [w774 w776]
              disable-tunnel: w766 -> [w773 w775]
              disable-tunnel: w762 -> [w772 _]
              disable-tunnel: [w771 w776] -> w761
              disable-tunnel: [w770 w775] -> w758
              frame Enabled {
                n141 = property class="SamplerPluginsBase.lvclass"(reference=w774, error in=w773, "Accessors:MultiPointParams"=w772) -> (reference out=w771:refnum<class "SamplerPluginsBase.lvclass">, error out=w770:errorcluster)
              }
              frame Disabled {
              }
            }
            n142 = call "StatusUpdate.vi"("error in (no error)"=w758, "Status"="Received Multi-Point Params" ("input 3"), "ModuleID"=w759) -> ("error out"=w764:errorcluster)  [unwired: 8 in]
          }
          frame "WriteCorrFactors" {
            n143 = Variant To Data(error in=w788, type=T10 {"MagCorr"=[], "DlyCorr"=[]} ("ReadMultiPointParams"), Variant=w789) -> (data=w782:T10, error out=w786:errorcluster)
            n144 = property class="ModuleAdmin.lvclass"(reference=w785) -> (reference out=w780:refnum<class "ModuleAdmin.lvclass">, "Accessors:Module ID"=w779:i32)  [unwired: 1 in, 1 out]
            n145 = property class="SamplerPluginsBase.lvclass"(reference=w787, error in=w786, "Accessors:CorrectionFactors"=w782) -> (reference out=w781:refnum<class "SamplerPluginsBase.lvclass">, error out=w778:errorcluster)
            n146 = call "StatusUpdate.vi"("error in (no error)"=w778, "Status"="Received CorrectionFactors" ("input 3"), "ModuleID"=w779) -> ("error out"=w784:errorcluster)  [unwired: 8 in]
          }
          frame "WriteMultiPointConfig" {
            n147 = Variant To Data(error in=w801, type=T8 {"iTriggerCount"=0, "iSampleCount"=0, "eSampleClock"=0, "dSampleInterval"=0.0} ("ReadMultiPointParams"), Variant=w802) -> (data=w795:T8, error out=w799:errorcluster)
            n148 = property class="ModuleAdmin.lvclass"(reference=w798) -> (reference out=w793:refnum<class "ModuleAdmin.lvclass">, "Accessors:Module ID"=w792:i32)  [unwired: 1 in, 1 out]
            n149 = property class="SamplerPluginsBase.lvclass"(reference=w800, error in=w799, "Accessors:ConfigMultiPointParams"=w795) -> (reference out=w794:refnum<class "SamplerPluginsBase.lvclass">, error out=w791:errorcluster)
            n150 = call "StatusUpdate.vi"("error in (no error)"=w791, "Status"="Received Multi-Point Params" ("input 3"), "ModuleID"=w792) -> ("error out"=w797:errorcluster)  [unwired: 8 in]
          }
          frame "ReadMultiPointParams" {
            n151 = property class="SamplerPluginsBase.lvclass"(reference=w812) -> (reference out=w805:refnum<class "SamplerPluginsBase.lvclass">, "Accessors:MultiPointParams"=w809:T9)  [unwired: 1 in, 1 out]
            n152 = property class="ModuleAdmin.lvclass"(reference=w810) -> (reference out=w806:refnum<class "ModuleAdmin.lvclass">, "Accessors:Module ID"=w807:i32)  [unwired: 1 in, 1 out]
            n153 = call "MultiPointParamBroadcast.vi"("error in (no error)"=w811, "MultiPointParams"=w809, "ModuleID"=w807) -> ("error out"=w808:errorcluster)  [unwired: 8 in]
            n154 = call "StatusUpdate.vi"("error in (no error)"=w808, "Status"="Transmitted MultiPoint Params", "ModuleID"=w807) -> ("error out"=w803:errorcluster)  [unwired: 8 in]
          }
          frame "ReadMultiPointConfig" {
            n155 = property class="SamplerPluginsBase.lvclass"(reference=w822) -> (reference out=w816:refnum<class "SamplerPluginsBase.lvclass">, "Accessors:ConfigMultiPointParams"=w813:T8)  [unwired: 1 in, 1 out]
            n156 = property class="ModuleAdmin.lvclass"(reference=w820) -> (reference out=w817:refnum<class "ModuleAdmin.lvclass">, "Accessors:Module ID"=w818:i32)  [unwired: 1 in, 1 out]
            n157 = call "MultiPointConfigBroadcast.vi"("error in (no error)"=w821, "MultiPointConfig"=w813, "ModuleID"=w818) -> ("error out"=w819:errorcluster)  [unwired: 8 in]
            n158 = call "StatusUpdate.vi"("error in (no error)"=w819, "Status"="Transmitted MultiPoint Config", "ModuleID"=w818) -> ("error out"=w814:errorcluster)  [unwired: 8 in]
          }
          frame "ReadCorrFactors" {
            n159 = property class="SamplerPluginsBase.lvclass"(reference=w832) -> (reference out=w826:refnum<class "SamplerPluginsBase.lvclass">, "Accessors:CorrectionFactors"=w823:T10)  [unwired: 1 in, 1 out]
            n160 = property class="ModuleAdmin.lvclass"(reference=w830) -> (reference out=w827:refnum<class "ModuleAdmin.lvclass">, "Accessors:Module ID"=w828:i32)  [unwired: 1 in, 1 out]
            n161 = call "CorrFactorsBroadcast.vi"("error in (no error)"=w831, "CorrectionFactors"=w823, "ModuleID"=w828) -> ("error out"=w829:errorcluster)  [unwired: 8 in]
            n162 = call "StatusUpdate.vi"("error in (no error)"=w829, "Status"="Transmitted CorrectionFactors", "ModuleID"=w828) -> ("error out"=w824:errorcluster)  [unwired: 8 in]
          }
          frame "WriteEvtSignal" {
            n163 = Variant To Data(error in=w843, type=dbl[][] [], Variant=w845) -> (data=w833:dbl[][], error out=w841:errorcluster)
            n164 = property class="ModuleAdmin.lvclass"(reference=w839) -> (reference out=w838:refnum<class "ModuleAdmin.lvclass">, "Accessors:Module ID"=w835:i32)  [unwired: 1 in, 1 out]
            n165 = call-dynamic "WriteEvtSignal.vi"("error in (no error)"=w841, "EvtSignal"=w833, "SamplerPluginsBase in"=w842) -> ("error out"=w837:errorcluster, "SamplerPluginsBase out"=w840:refnum<class "SamplerPluginsBase.lvclass">)  [unwired: 7 in]
            n166 = call "StatusUpdate.vi"("error in (no error)"=w837, "Status"="Received Waveform", "ModuleID"=w835) -> ("error out"=w836:errorcluster)  [unwired: 8 in]
          }
          frame "ShowPanel" {
            n167 = Variant To Data(error in=w849, type=TRUE, Variant=w850) -> (data=w856:bool, error out=w853:errorcluster)
            n168 = Select(t=T4."Standard" ("Front Panel Window:State"), s=w856, f=T4."Hidden" ("Front Panel Window:State")) -> (s? t:f=w857:T4)
            n169 = property class="VI"(error in=w853, "FP.State"=w857) -> (error out=w851:errorcluster)  [unwired: 1 in, 1 out]
            n170 = property class="ModuleAdmin.lvclass"(reference=w848, "Accessors:ShowPanel_"=w856) -> (reference out=w847:refnum<class "ModuleAdmin.lvclass">)  [unwired: 1 in, 1 out]
          }
        }
        n171 = call-dynamic "DisplayProperties.vi"("Class In"=w359) -> ("Class out"=w358:refnum<class "SamplerPluginsBase.lvclass">)  [unwired: 10 in]
        n172 = call "ErrorHandler.vi"("error in (no error)"=w362, "MessageQueue"=w361) -> ("error out"=w363:errorcluster)  [unwired: 8 in, 1 out]
      }
      n173 = while {
        tunnel: w33 -> [w36]
        shift-right: [w40] -> w25
        shift-left: w31 -> [w41]
        tunnel: w30 -> [w39]
        tunnel: [w37] -> w26
        stop <- w42 stop-if-true
        # "Event Handler Loop"
        n174 = event shown="[13] <SamplerRequests.FetchRequest>: User Event" {
          selector: w41 -> [_ _ _ _ _ _ _ _ _ _ _ _ _ _ _ _ _ _ _ _ _ _ _ _ _ _ _ _ _ _ _]
          dyn-events: [_ _ _ _ _ _ _ _ _ _ _ _ _ _ _ _ _ _ _ _ _ _ _ _ _ _ _ _ _ _ _] -> w40
          timeout: _ -> [_ _ _ _ _ _ _ _ _ _ _ _ _ _ _ _ _ _ _ _ _ _ _ _ _ _ _ _ _ _ _]
          tunnel: w36 -> [w46 w68 w71 w82 w91 w100 w110 w120 w130 w140 w150 w160 w170 w180 w190 w200 w210 w220 w230 w240 w250 w259 w268 w278 w288 w298 w308 w318 w328 w338 w349]
          tunnel: [w45 TRUE _ _ _ _ _ _ _ _ _ _ _ _ _ _ _ _ _ _ _ _ _ _ _ _ _ _ _ _ _] -> w42
          tunnel: w39 -> [w49 w62 w70 w86 w95 w104 w114 w124 w134 w144 w154 w164 w174 w184 w194 w204 w214 w224 w234 w244 w254 w263 w272 w282 w292 w302 w312 w322 w332 w342 w352]
          tunnel: [w44 w66 w69 w83 w92 w101 w111 w121 w131 w141 w151 w161 w171 w181 w191 w201 w211 w221 w231 w241 w251 w260 w269 w279 w289 w299 w309 w319 w329 w339 w347] -> w38
          event User Event {
            # "Called from another module or the QMH"
            n175 = event-data() -> ("ModuleID"=w47:i32, "Data"=w43:variant)  [unwired: 1 in]
            n176 = call <userlib>:"AddressedToThisModule.vi"("ModuleID"=w47, "ModuleAdmin"=w49) -> ("AddressedToThisInstance?"=w48:bool)  [unwired: 8 in, 1 out]
            n177 = case shown="True" w48 {
              tunnel: w47 -> [_ _]
              tunnel: w46 -> [_ w55]
              tunnel: [FALSE TRUE] -> w45
              tunnel: [_ w53] -> w44
              tunnel: w43 -> [_ w51]
              frame False {
                # "The stop request was for a different module"
              }
              frame True {
                # "The stop request was for this module"
                n178 = call "Enqueue.vi"("Message Data"=w51, "Message"="Exit", "MessageQueue"=w55) -> ("error out"=w53:errorcluster)  [unwired: 7 in, 1 out]
              }
            }
          }
          event Panel Close? {
            # "Hide on external launch"
            # "Discard the event so the QMH can complete"
            # "Called from another module or the QMH"
            n179 = event-data() -> ()  [unwired: 1 in, 1 out]
            n180 = property class="ModuleAdmin.lvclass"(reference=w62) -> ("Accessors:External Launch"=w57:bool)  [unwired: 1 in, 2 out]
            n181 = Bundle By Name(cluster=T3 {"Exit via Stop Module Req?"=FALSE, "Wait for Module to stop?"=FALSE, "ModuleAdmin"=refnum} ("Stop Argument"), "Wait for Module to stop?"=FALSE, "Exit via Stop Module Req?"=TRUE) -> (w63:T3)
            n182 = Select(t="HidePanel", s=w57, f="Exit" ("Message")) -> (s? t:f=w59:string)
            n183 = call "Enqueue.vi"("Message Data"=w63, "Message"=w59, "MessageQueue"=w68) -> ("error out"=w66:errorcluster)  [unwired: 7 in, 1 out]
            n184 = event-data("Discard?"=TRUE) -> ()  [unwired: 1 in, 1 out]
          }
          event User Event {
            n185 = event-data() -> ("ModuleID"=w72:i32, "Data"=w73:variant)  [unwired: 1 in]
            n186 = call <userlib>:"AddressedToThisModule.vi"("ModuleID"=w72, "ModuleAdmin"=w70) -> ("AddressedToThisInstance?"=w74:bool)  [unwired: 8 in, 1 out]
            n187 = case shown="True" w74 {
              tunnel: w72 -> [_ _]
              tunnel: w71 -> [_ w80]
              tunnel: [FALSE TRUE] -> _
              tunnel: [_ w78] -> w69
              tunnel: w73 -> [_ w76]
              frame False {
                # "The stop request was for a different module"
              }
              frame True {
                # "The stop request was for this module"
                n188 = call "Enqueue.vi"("Message Data"=w76, "Message"="GetPathToINI", "MessageQueue"=w80) -> ("error out"=w78:errorcluster)  [unwired: 7 in, 1 out]
              }
            }
          }
          event User Event {
            n189 = event-data() -> ("ModuleID"=w85:i32, "Data"=w81:variant)  [unwired: 1 in]
            n190 = call <userlib>:"AddressedToThisModule.vi"("ModuleID"=w85, "ModuleAdmin"=w86) -> ("AddressedToThisInstance?"=w84:bool)  [unwired: 8 in, 1 out]
            n191 = case shown="True" w84 {
              tunnel: [_ w87] -> w83
              tunnel: w82 -> [_ w90]
              tunnel: w81 -> [_ w88]
              frame False {
              }
              frame True {
                n192 = call "Enqueue.vi"("Message Data"=w88, "Message"="LoadPlugin", "MessageQueue"=w90) -> ("error out"=w87:errorcluster)  [unwired: 7 in, 1 out]
              }
            }
          }
          event User Event {
            n193 = event-data() -> ("ModuleID"=w94:i32)  [unwired: 1 in]
            n194 = call <userlib>:"AddressedToThisModule.vi"("ModuleID"=w94, "ModuleAdmin"=w95) -> ("AddressedToThisInstance?"=w93:bool)  [unwired: 8 in, 1 out]
            n195 = case shown="True" w93 {
              tunnel: [_ w96] -> w92
              tunnel: w91 -> [_ w98]
              frame False {
              }
              frame True {
                n196 = call "Enqueue.vi"("Message"="ConfigDialog", "MessageQueue"=w98) -> ("error out"=w96:errorcluster)  [unwired: 8 in, 1 out]
              }
            }
          }
          event User Event {
            n197 = event-data() -> ("ModuleID"=w103:i32, "Data"=w99:variant)  [unwired: 1 in]
            n198 = call <userlib>:"AddressedToThisModule.vi"("ModuleID"=w103, "ModuleAdmin"=w104) -> ("AddressedToThisInstance?"=w102:bool)  [unwired: 8 in, 1 out]
            n199 = case shown="True" w102 {
              tunnel: [_ w105] -> w101
              tunnel: w100 -> [_ w108]
              tunnel: w99 -> [_ w106]
              frame False {
              }
              frame True {
                n200 = call "Enqueue.vi"("Message Data"=w106, "Message"="Reset", "MessageQueue"=w108) -> ("error out"=w105:errorcluster)  [unwired: 7 in, 1 out]
              }
            }
          }
          event User Event {
            n201 = event-data() -> ("ModuleID"=w113:i32, "Data"=w109:variant)  [unwired: 1 in]
            n202 = call <userlib>:"AddressedToThisModule.vi"("ModuleID"=w113, "ModuleAdmin"=w114) -> ("AddressedToThisInstance?"=w112:bool)  [unwired: 8 in, 1 out]
            n203 = case shown="True" w112 {
              tunnel: [_ w115] -> w111
              tunnel: w110 -> [_ w118]
              tunnel: w109 -> [_ w116]
              frame False {
              }
              frame True {
                n204 = call "Enqueue.vi"("Message Data"=w116, "Message"="Abort", "MessageQueue"=w118) -> ("error out"=w115:errorcluster)  [unwired: 7 in, 1 out]
              }
            }
          }
          event User Event {
            n205 = event-data() -> ("ModuleID"=w123:i32, "Data"=w119:variant)  [unwired: 1 in]
            n206 = call <userlib>:"AddressedToThisModule.vi"("ModuleID"=w123, "ModuleAdmin"=w124) -> ("AddressedToThisInstance?"=w122:bool)  [unwired: 8 in, 1 out]
            n207 = case shown="True" w122 {
              tunnel: [_ w125] -> w121
              tunnel: w120 -> [_ w128]
              tunnel: w119 -> [_ w126]
              frame False {
              }
              frame True {
                n208 = call "Enqueue.vi"("Message Data"=w126, "Message"="InitializeDevice", "MessageQueue"=w128) -> ("error out"=w125:errorcluster)  [unwired: 7 in, 1 out]
              }
            }
          }
          event User Event {
            n209 = event-data() -> ("ModuleID"=w133:i32, "Data"=w129:variant)  [unwired: 1 in]
            n210 = call <userlib>:"AddressedToThisModule.vi"("ModuleID"=w133, "ModuleAdmin"=w134) -> ("AddressedToThisInstance?"=w132:bool)  [unwired: 8 in, 1 out]
            n211 = case shown="True" w132 {
              tunnel: [_ w135] -> w131
              tunnel: w130 -> [_ w138]
              tunnel: w129 -> [_ w136]
              frame False {
              }
              frame True {
                n212 = call "Enqueue.vi"("Message Data"=w136, "Message"="ConfigMeasurement", "MessageQueue"=w138) -> ("error out"=w135:errorcluster)  [unwired: 7 in, 1 out]
              }
            }
          }
          event User Event {
            n213 = event-data() -> ("ModuleID"=w143:i32, "Data"=w139:variant)  [unwired: 1 in]
            n214 = call <userlib>:"AddressedToThisModule.vi"("ModuleID"=w143, "ModuleAdmin"=w144) -> ("AddressedToThisInstance?"=w142:bool)  [unwired: 8 in, 1 out]
            n215 = case shown="True" w142 {
              tunnel: [_ w145] -> w141
              tunnel: w140 -> [_ w148]
              tunnel: w139 -> [_ w146]
              frame False {
              }
              frame True {
                n216 = call "Enqueue.vi"("Message Data"=w146, "Message"="ConfigTrigger", "MessageQueue"=w148) -> ("error out"=w145:errorcluster)  [unwired: 7 in, 1 out]
              }
            }
          }
          event User Event {
            n217 = event-data() -> ("ModuleID"=w153:i32, "Data"=w149:variant)  [unwired: 1 in]
            n218 = call <userlib>:"AddressedToThisModule.vi"("ModuleID"=w153, "ModuleAdmin"=w154) -> ("AddressedToThisInstance?"=w152:bool)  [unwired: 8 in, 1 out]
            n219 = case shown="True" w152 {
              tunnel: [_ w155] -> w151
              tunnel: w150 -> [_ w158]
              tunnel: w149 -> [_ w156]
              frame False {
              }
              frame True {
                n220 = call "Enqueue.vi"("Message Data"=w156, "Message"="ConfigACBandwidth", "MessageQueue"=w158) -> ("error out"=w155:errorcluster)  [unwired: 7 in, 1 out]
              }
            }
          }
          event User Event {
            n221 = event-data() -> ("ModuleID"=w163:i32, "Data"=w159:variant)  [unwired: 1 in]
            n222 = call <userlib>:"AddressedToThisModule.vi"("ModuleID"=w163, "ModuleAdmin"=w164) -> ("AddressedToThisInstance?"=w162:bool)  [unwired: 8 in, 1 out]
            n223 = case shown="True" w162 {
              tunnel: [_ w165] -> w161
              tunnel: w160 -> [_ w168]
              tunnel: w159 -> [_ w166]
              frame False {
              }
              frame True {
                n224 = call "Enqueue.vi"("Message Data"=w166, "Message"="ConfigFreqVoltRange", "MessageQueue"=w168) -> ("error out"=w165:errorcluster)  [unwired: 7 in, 1 out]
              }
            }
          }
          event User Event {
            n225 = event-data() -> ("ModuleID"=w173:i32, "Data"=w169:variant)  [unwired: 1 in]
            n226 = call <userlib>:"AddressedToThisModule.vi"("ModuleID"=w173, "ModuleAdmin"=w174) -> ("AddressedToThisInstance?"=w172:bool)  [unwired: 8 in, 1 out]
            n227 = case shown="True" w172 {
              tunnel: [_ w175] -> w171
              tunnel: w170 -> [_ w178]
              tunnel: w169 -> [_ w176]
              frame False {
              }
              frame True {
                n228 = call "Enqueue.vi"("Message Data"=w176, "Message"="Read", "MessageQueue"=w178) -> ("error out"=w175:errorcluster)  [unwired: 7 in, 1 out]
              }
            }
          }
          event User Event {
            n229 = event-data() -> ("ModuleID"=w183:i32, "Data"=w179:variant)  [unwired: 1 in]
            n230 = call <userlib>:"AddressedToThisModule.vi"("ModuleID"=w183, "ModuleAdmin"=w184) -> ("AddressedToThisInstance?"=w182:bool)  [unwired: 8 in, 1 out]
            n231 = case shown="True" w182 {
              tunnel: [_ w185] -> w181
              tunnel: w180 -> [_ w188]
              tunnel: w179 -> [_ w186]
              frame False {
              }
              frame True {
                n232 = call "Enqueue.vi"("Message Data"=w186, "Message"="Fetch", "MessageQueue"=w188) -> ("error out"=w185:errorcluster)  [unwired: 7 in, 1 out]
              }
            }
          }
          event User Event {
            n233 = event-data() -> ("ModuleID"=w193:i32, "Data"=w189:variant)  [unwired: 1 in]
            n234 = call <userlib>:"AddressedToThisModule.vi"("ModuleID"=w193, "ModuleAdmin"=w194) -> ("AddressedToThisInstance?"=w192:bool)  [unwired: 8 in, 1 out]
            n235 = case shown="True" w192 {
              tunnel: [_ w195] -> w191
              tunnel: w190 -> [_ w198]
              tunnel: w189 -> [_ w196]
              frame False {
              }
              frame True {
                n236 = call "Enqueue.vi"("Message Data"=w196, "Message"="Initiate", "MessageQueue"=w198) -> ("error out"=w195:errorcluster)  [unwired: 7 in, 1 out]
              }
            }
          }
          event User Event {
            n237 = event-data() -> ("ModuleID"=w203:i32, "Data"=w199:variant)  [unwired: 1 in]
            n238 = call <userlib>:"AddressedToThisModule.vi"("ModuleID"=w203, "ModuleAdmin"=w204) -> ("AddressedToThisInstance?"=w202:bool)  [unwired: 8 in, 1 out]
            n239 = case shown="True" w202 {
              tunnel: [_ w205] -> w201
              tunnel: w200 -> [_ w208]
              tunnel: w199 -> [_ w206]
              frame False {
              }
              frame True {
                n240 = call "Enqueue.vi"("Message Data"=w206, "Message"="GetReading", "MessageQueue"=w208) -> ("error out"=w205:errorcluster)  [unwired: 7 in, 1 out]
              }
            }
          }
          event User Event {
            n241 = event-data() -> ("ModuleID"=w213:i32, "Data"=w209:variant)  [unwired: 1 in]
            n242 = call <userlib>:"AddressedToThisModule.vi"("ModuleID"=w213, "ModuleAdmin"=w214) -> ("AddressedToThisInstance?"=w212:bool)  [unwired: 8 in, 1 out]
            n243 = case shown="True" w212 {
              tunnel: [_ w215] -> w211
              tunnel: w210 -> [_ w218]
              tunnel: w209 -> [_ w216]
              frame False {
              }
              frame True {
                n244 = call "Enqueue.vi"("Message Data"=w216, "Message"="IsOverRange", "MessageQueue"=w218) -> ("error out"=w215:errorcluster)  [unwired: 7 in, 1 out]
              }
            }
          }
          event User Event {
            n245 = event-data() -> ("ModuleID"=w223:i32, "Data"=w219:variant)  [unwired: 1 in]
            n246 = call <userlib>:"AddressedToThisModule.vi"("ModuleID"=w223, "ModuleAdmin"=w224) -> ("AddressedToThisInstance?"=w222:bool)  [unwired: 8 in, 1 out]
            n247 = case shown="True" w222 {
              tunnel: [_ w225] -> w221
              tunnel: w220 -> [_ w228]
              tunnel: w219 -> [_ w226]
              frame False {
              }
              frame True {
                n248 = call "Enqueue.vi"("Message Data"=w226, "Message"="ConfigMeasCompDest", "MessageQueue"=w228) -> ("error out"=w225:errorcluster)  [unwired: 7 in, 1 out]
              }
            }
          }
          event User Event {
            n249 = event-data() -> ("ModuleID"=w233:i32, "Data"=w229:variant)  [unwired: 1 in]
            n250 = call <userlib>:"AddressedToThisModule.vi"("ModuleID"=w233, "ModuleAdmin"=w234) -> ("AddressedToThisInstance?"=w232:bool)  [unwired: 8 in, 1 out]
            n251 = case shown="True" w232 {
              tunnel: [_ w235] -> w231
              tunnel: w230 -> [_ w238]
              tunnel: w229 -> [_ w236]
              frame False {
              }
              frame True {
                n252 = call "Enqueue.vi"("Message Data"=w236, "Message"="ConfigMultiPoint", "MessageQueue"=w238) -> ("error out"=w235:errorcluster)  [unwired: 7 in, 1 out]
              }
            }
          }
          event User Event {
            n253 = event-data() -> ("ModuleID"=w243:i32, "Data"=w239:variant)  [unwired: 1 in]
            n254 = call <userlib>:"AddressedToThisModule.vi"("ModuleID"=w243, "ModuleAdmin"=w244) -> ("AddressedToThisInstance?"=w242:bool)  [unwired: 8 in, 1 out]
            n255 = case shown="True" w242 {
              tunnel: [_ w245] -> w241
              tunnel: w240 -> [_ w248]
              tunnel: w239 -> [_ w246]
              frame False {
              }
              frame True {
                n256 = call "Enqueue.vi"("Message Data"=w246, "Message"="InitiateMultiPoint", "MessageQueue"=w248) -> ("error out"=w245:errorcluster)  [unwired: 7 in, 1 out]
              }
            }
          }
          event User Event {
            n257 = event-data() -> ("ModuleID"=w253:i32, "Data"=w249:variant)  [unwired: 1 in]
            n258 = call <userlib>:"AddressedToThisModule.vi"("ModuleID"=w253, "ModuleAdmin"=w254) -> ("AddressedToThisInstance?"=w252:bool)  [unwired: 8 in, 1 out]
            n259 = case shown="True" w252 {
              tunnel: [_ w255] -> w251
              tunnel: w250 -> [_ w258]
              tunnel: w249 -> [_ w256]
              frame False {
              }
              frame True {
                n260 = call "Enqueue.vi"("Message Data"=w256, "Message"="FetchMultiPoint", "MessageQueue"=w258) -> ("error out"=w255:errorcluster)  [unwired: 7 in, 1 out]
              }
            }
          }
          event User Event {
            n261 = event-data() -> ("ModuleID"=w262:i32)  [unwired: 1 in]
            n262 = call <userlib>:"AddressedToThisModule.vi"("ModuleID"=w262, "ModuleAdmin"=w263) -> ("AddressedToThisInstance?"=w261:bool)  [unwired: 8 in, 1 out]
            n263 = case shown="True" w261 {
              tunnel: [_ w264] -> w260
              tunnel: w259 -> [_ w266]
              frame False {
              }
              frame True {
                n264 = call "Enqueue.vi"("Message"="ReadMultiPoint", "MessageQueue"=w266) -> ("error out"=w264:errorcluster)  [unwired: 8 in, 1 out]
              }
            }
          }
          event User Event {
            n265 = event-data() -> ("ModuleID"=w271:i32, "Data"=w267:variant)  [unwired: 1 in]
            n266 = call <userlib>:"AddressedToThisModule.vi"("ModuleID"=w271, "ModuleAdmin"=w272) -> ("AddressedToThisInstance?"=w270:bool)  [unwired: 8 in, 1 out]
            n267 = case shown="True" w270 {
              tunnel: [_ w273] -> w269
              tunnel: w268 -> [_ w276]
              tunnel: w267 -> [_ w274]
              frame False {
              }
              frame True {
                n268 = call "Enqueue.vi"("Message Data"=w274, "Message"="WriteMultiPointParams", "MessageQueue"=w276) -> ("error out"=w273:errorcluster)  [unwired: 7 in, 1 out]
              }
            }
          }
          event User Event {
            n269 = event-data() -> ("ModuleID"=w281:i32, "Data"=w277:variant)  [unwired: 1 in]
            n270 = call <userlib>:"AddressedToThisModule.vi"("ModuleID"=w281, "ModuleAdmin"=w282) -> ("AddressedToThisInstance?"=w280:bool)  [unwired: 8 in, 1 out]
            n271 = case shown="True" w280 {
              tunnel: [_ w283] -> w279
              tunnel: w278 -> [_ w286]
              tunnel: w277 -> [_ w284]
              frame False {
              }
              frame True {
                n272 = call "Enqueue.vi"("Message Data"=w284, "Message"="ReadMultiPointParams", "MessageQueue"=w286) -> ("error out"=w283:errorcluster)  [unwired: 7 in, 1 out]
              }
            }
          }
          event User Event {
            n273 = event-data() -> ("ModuleID"=w291:i32, "Data"=w287:variant)  [unwired: 1 in]
            n274 = call <userlib>:"AddressedToThisModule.vi"("ModuleID"=w291, "ModuleAdmin"=w292) -> ("AddressedToThisInstance?"=w290:bool)  [unwired: 8 in, 1 out]
            n275 = case shown="True" w290 {
              tunnel: [_ w293] -> w289
              tunnel: w288 -> [_ w296]
              tunnel: w287 -> [_ w294]
              frame False {
              }
              frame True {
                n276 = call "Enqueue.vi"("Message Data"=w294, "Message"="WriteMultiPointConfig", "MessageQueue"=w296) -> ("error out"=w293:errorcluster)  [unwired: 7 in, 1 out]
              }
            }
          }
          event User Event {
            n277 = event-data() -> ("ModuleID"=w301:i32, "Data"=w297:variant)  [unwired: 1 in]
            n278 = call <userlib>:"AddressedToThisModule.vi"("ModuleID"=w301, "ModuleAdmin"=w302) -> ("AddressedToThisInstance?"=w300:bool)  [unwired: 8 in, 1 out]
            n279 = case shown="True" w300 {
              tunnel: [_ w303] -> w299
              tunnel: w298 -> [_ w306]
              tunnel: w297 -> [_ w304]
              frame False {
              }
              frame True {
                n280 = call "Enqueue.vi"("Message Data"=w304, "Message"="ReadMultiPointConfig", "MessageQueue"=w306) -> ("error out"=w303:errorcluster)  [unwired: 7 in, 1 out]
              }
            }
          }
          event User Event {
            n281 = event-data() -> ("ModuleID"=w311:i32, "Data"=w307:variant)  [unwired: 1 in]
            n282 = call <userlib>:"AddressedToThisModule.vi"("ModuleID"=w311, "ModuleAdmin"=w312) -> ("AddressedToThisInstance?"=w310:bool)  [unwired: 8 in, 1 out]
            n283 = case shown="True" w310 {
              tunnel: [_ w313] -> w309
              tunnel: w308 -> [_ w316]
              tunnel: w307 -> [_ w314]
              frame False {
              }
              frame True {
                n284 = call "Enqueue.vi"("Message Data"=w314, "Message"="ReadCorrFactors", "MessageQueue"=w316) -> ("error out"=w313:errorcluster)  [unwired: 7 in, 1 out]
              }
            }
          }
          event User Event {
            n285 = event-data() -> ("ModuleID"=w321:i32, "Data"=w317:variant)  [unwired: 1 in]
            n286 = call <userlib>:"AddressedToThisModule.vi"("ModuleID"=w321, "ModuleAdmin"=w322) -> ("AddressedToThisInstance?"=w320:bool)  [unwired: 8 in, 1 out]
            n287 = case shown="True" w320 {
              tunnel: [_ w323] -> w319
              tunnel: w318 -> [_ w326]
              tunnel: w317 -> [_ w324]
              frame False {
              }
              frame True {
                n288 = call "Enqueue.vi"("Message Data"=w324, "Message"="WriteCorrFactors", "MessageQueue"=w326) -> ("error out"=w323:errorcluster)  [unwired: 7 in, 1 out]
              }
            }
          }
          event User Event {
            n289 = event-data() -> ("ModuleID"=w331:i32, "Data"=w327:variant)  [unwired: 1 in]
            n290 = call <userlib>:"AddressedToThisModule.vi"("ModuleID"=w331, "ModuleAdmin"=w332) -> ("AddressedToThisInstance?"=w330:bool)  [unwired: 8 in, 1 out]
            n291 = case shown="True" w330 {
              tunnel: [_ w333] -> w329
              tunnel: w328 -> [_ w336]
              tunnel: w327 -> [_ w334]
              frame False {
              }
              frame True {
                n292 = call "Enqueue.vi"("Message Data"=w334, "Message"="GetMultiPointReading", "MessageQueue"=w336) -> ("error out"=w333:errorcluster)  [unwired: 7 in, 1 out]
              }
            }
          }
          event User Event {
            n293 = event-data() -> ("ModuleID"=w341:i32, "Data"=w337:variant)  [unwired: 1 in]
            n294 = call <userlib>:"AddressedToThisModule.vi"("ModuleID"=w341, "ModuleAdmin"=w342) -> ("AddressedToThisInstance?"=w340:bool)  [unwired: 8 in, 1 out]
            n295 = case shown="True" w340 {
              tunnel: [_ w343] -> w339
              tunnel: w338 -> [_ w346]
              tunnel: w337 -> [_ w344]
              frame False {
              }
              frame True {
                n296 = call "Enqueue.vi"("Message Data"=w344, "Message"="WriteEvtSignal", "MessageQueue"=w346) -> ("error out"=w343:errorcluster)  [unwired: 7 in, 1 out]
              }
            }
          }
          event User Event {
            n297 = event-data() -> ("ModuleID"=w351:i32, "Data"=w348:variant)  [unwired: 1 in]
            n298 = call <userlib>:"AddressedToThisModule.vi"("ModuleID"=w351, "ModuleAdmin"=w352) -> ("AddressedToThisInstance?"=w350:bool)  [unwired: 8 in, 1 out]
            n299 = case shown="True" w350 {
              tunnel: w349 -> [_ w356]
              tunnel: w348 -> [_ w355]
              tunnel: [_ w353] -> w347
              frame False {
              }
              frame True {
                n300 = call "Enqueue.vi"("Message Data"=w355, "Message"="ShowPanel", "MessageQueue"=w356) -> ("error out"=w353:errorcluster)  [unwired: 7 in, 1 out]
              }
            }
          }
        }
        n301 = call "ErrorHandler.vi"("error in (no error)"=w38, "MessageQueue"=w36) -> ("error out"=w37:errorcluster)  [unwired: 8 in, 1 out]
      }
    }
    frame Error {
      n302 = property class="ModuleAdmin.lvclass"(reference=w863) -> (reference out=w861:refnum<class "ModuleAdmin.lvclass">, "Accessors:CloneRegRef"=w860:refnum<data-value>, "Accessors:Module ID"=w859:i32)  [unwired: 1 in, 1 out]
      n303 = call <userlib>:"Remove.vi"("Module ID"=w859, "CloneRegRef"=w860) -> ("error out"=w865:errorcluster)  [unwired: 7 in, 2 out]
      n304 = flat-sequence {
        tunnel: w866 -> [w869]
        tunnel: w865 -> [_]
        tunnel: [w867] -> w864
        frame #0 {
          w868 = T13 2 items=["no dialog", "OK message", "continue or stop message", "OK message + warnings", "continue/stop + warnings"] ("type of dialog (OK msg:1)")
          n305 = call <vilib>:"Simple Error Handler.vi"("type of dialog (OK msg:1)"=w868, "error in (no error)"=w869) -> ("error out"=w867:errorcluster)  [unwired: 3 in, 4 out]
        }
      }
    }
  }
  n306 = Unregister For Events(event registration refnum=w4, error in=w5) -> (error out=w2:errorcluster)
  n307 = call "DestroyClone.vi"("error in (no error)"=w12, "Exit via Stop Module Req?"=w8, "Wait for Module to stop?"=w9, "ModuleAdmin"=w10) -> ("error out"=w11:errorcluster, "External Launch"=w7:bool)  [unwired: 5 in, 1 out]
  n308 = Release Queue(queue=w17, error in (no error)=w11) -> (error out=w6:errorcluster)  [unwired: 1 in, 2 out]
  n309 = Merge Errors(w2, w6) -> (w3:errorcluster)
  "error out" <- w3
  n310 = case shown="True" w7 {
    tunnel: w3 -> [_ w871]
    frame False {
    }
    frame True {
      n311 = control-ref of="This VI"() -> (w870:refnum<vi>)
      n312 = case shown="Error" w871 {
        tunnel: w870 -> [w872 w873]
        frame No Error {
          n313 = invoke class="VI" method="FP.Close"(reference=w872) -> ()  [unwired: 2 in, 3 out]
        }
        frame Error {
          n314 = invoke class="VI" method="FP.Open"(reference=w873, "Activate"=TRUE ("Activate?")) -> ()  [unwired: 3 in, 5 out]
        }
      }
    }
  }
